vi "Set 135 Interval via GPIB.vi"(3 "error in":T1, 4 "Hidden Controls (in)":T2 {"Prev Sampling Interval" format="%.1f"; "Prev Lo Setpoint" format="%.1f"; "Prev Hi Setpoint" format="%.1f"; "Prev Sensor Length" format="%.1f"; "Helium Level (cm)" format="%.1f"}, 5 "Configuration (in)":T3={"Sensor Length (cm)"=100.0, "Hi Setpoint (cm)"=80.0, "Lo Setpoint (cm)"=20.0, "Sampling Interval (min)"=1.0} {"Sampling Interval (min)" min=0 max=600 format="%.1f"; "Lo Setpoint (cm)" min=0 max=203.2 format="%.1f"; "Hi Setpoint (cm)" min=0 max=203.2 format="%.1f"; "Sensor Length (cm)" min=1 max=203.2 format="%.1f"}, 6 "GPIB Setup":cluster{"GPIB address":i16, "GPIB bus":i16}={"GPIB address"=1, "GPIB bus"=0}) -> (0 "error out":T1, 1 "Hidden Controls (out)":T2 {"Prev Sampling Interval" format="%.1f"; "Prev Lo Setpoint" format="%.1f"; "Prev Hi Setpoint" format="%.1f"; "Prev Sensor Length" format="%.1f"; "Helium Level (cm)" format="%.1f"}, 2 "Configuration (out)":T3={"Sensor Length (cm)"=100.0, "Hi Setpoint (cm)"=80.0, "Lo Setpoint (cm)"=20.0, "Sampling Interval (min)"=1.0} {"Sampling Interval (min)" min=0 max=600 format="%.1f"; "Lo Setpoint (cm)" min=0 max=203.2 format="%.1f"; "Hi Setpoint (cm)" min=0 max=203.2 format="%.1f"; "Sensor Length (cm)" min=1 max=203.2 format="%.1f"})   [LabVIEW 2019]
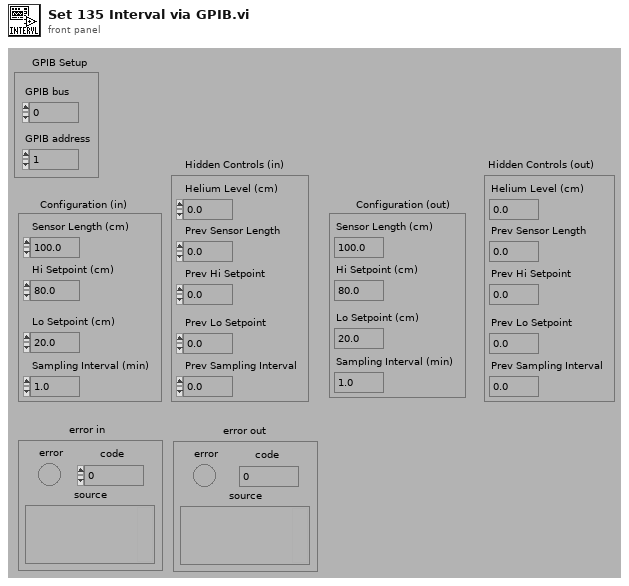
[diagram p1: front panel]
types:
  T1 = cluster{"error":bool, "code":i32, "source":string}
  T2 = cluster{"Helium Level (cm)":sgl, "Prev Sensor Length":sgl, "Prev Hi Setpoint":sgl, "Prev Lo Setpoint":sgl, "Prev Sampling Interval":sgl}
  T3 = cluster{"Sensor Length (cm)":sgl, "Hi Setpoint (cm)":sgl, "Lo Setpoint (cm)":sgl, "Sampling Interval (min)":sgl}
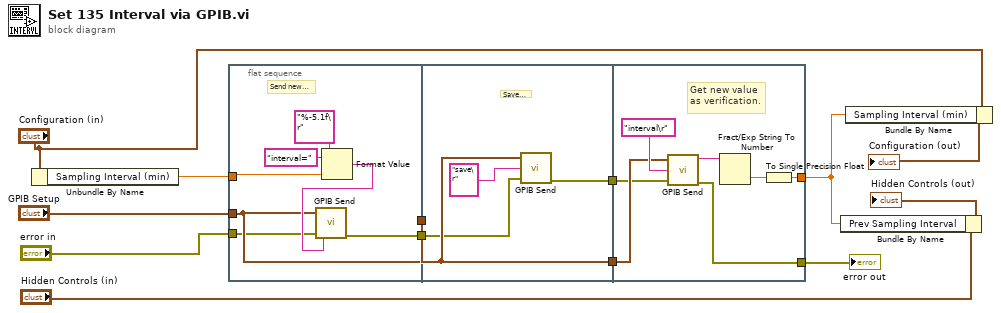
[diagram p0: block diagram]
diagram:
  n1 = Unbundle By Name("Configuration (in)") -> ("Sampling Interval (min)"=w8:sgl)
  n2 = flat-sequence {
    tunnel: "GPIB Setup" -> [w16]
    tunnel: [w16] -> w6
    tunnel: w8 -> [w19]
    tunnel: [w15] -> w2
    tunnel: "error in" -> [w14]
    tunnel: w6 -> [w23]
    tunnel: [w23] -> w5
    tunnel: [w22] -> w4
    tunnel: w2 -> [w21]
    tunnel: w5 -> [w28]
    tunnel: [w27] -> w12
    tunnel: w4 -> [w26]
    tunnel: [w25] -> w3
    frame #0 {
      # "Send new INTERVAL setting\nto instrument."
      n3 = Format Value(string ("")="interval=", format string="%-5.1f\r", value (0)=w19) -> (output string=w20:string)
      n4 = call "GPIB Send.vi"("GPIB Setup"=w16, "Input command"=w20, "error in"=w14) -> ("error out"=w15:T1)  [unwired: 3 out]
    }
    frame #1 {
      # "Save new setting."
      n5 = call "GPIB Send.vi"("GPIB Setup"=w23, "Input command"="save\r", "error in"=w21) -> ("error out"=w22:T1)  [unwired: 3 out]
    }
    frame #2 {
      # "Get new value\nas verification."
      n6 = call "GPIB Send.vi"("GPIB Setup"=w28, "Input command"="interval\r", "error in"=w26) -> ("Return string"=w30:string, "error out"=w25:T1)  [unwired: 2 out]
      n7 = Fract/Exp String To Number(string=w30) -> (number=w31:dbl)  [unwired: 3 in, 1 out]
      n8 = To Single Precision Float(number=w31) -> (single precision float=w27:sgl)
    }
  }
  n9 = Bundle By Name(cluster="Hidden Controls (in)", "Prev Sampling Interval"=w12) -> (→"Hidden Controls (out)":T2)
  n10 = Bundle By Name(cluster="Configuration (in)", "Sampling Interval (min)"=w12) -> (→"Configuration (out)":T3)
  "error out" <- w3
